vi "Test - DeviceManager - StartICL 1.vi"(8 "error in":errorcluster) -> (0 "error out":errorcluster, 3 "Pass":bool)   [LabVIEW 2023]
doc: "_____\nCreated using DQMH Event Scripter 7.0.0.1280."
uses:
  Source/Libraries/DeviceManager/DeviceManager.lvlib
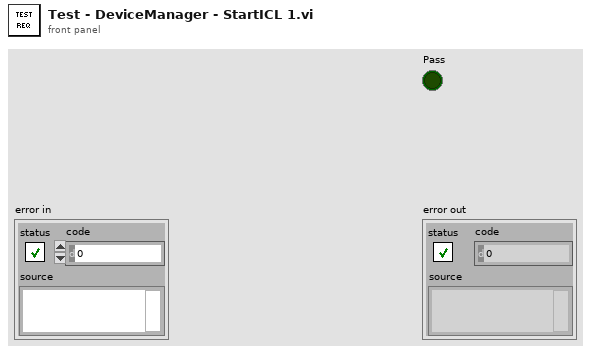
[diagram p1: front panel]
types:
  T1 = typedef "DeviceManager.lvlib/Broadcast Events--cluster.ctl" = cluster{"Module Did Init":refnum<user-event>, "Status Updated":refnum<user-event>, "Error Reported":refnum<user-event>, "Module Did Stop":refnum<user-event>, "Update Module Execution Status":refnum<user-event>}
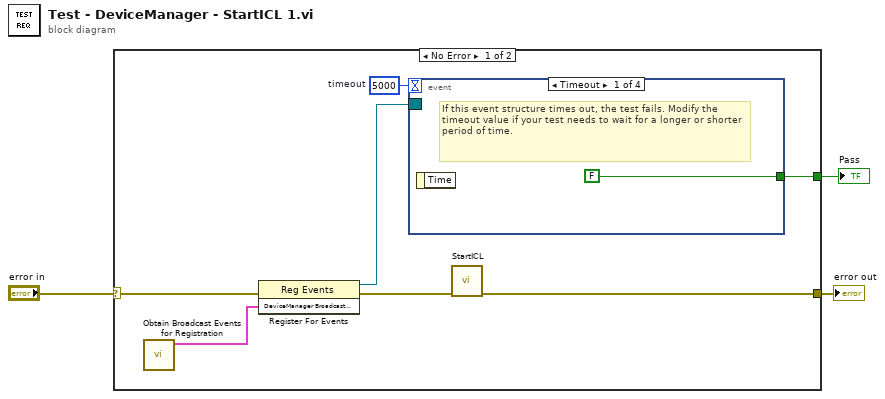
[diagram p0: block diagram]
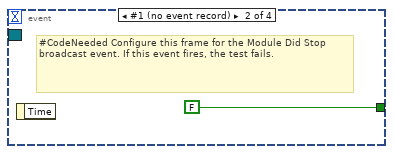
[diagram p2: hidden frame]
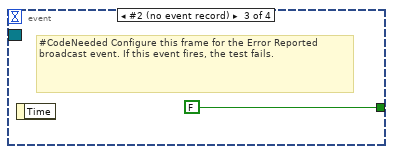
[diagram p3: hidden frame]
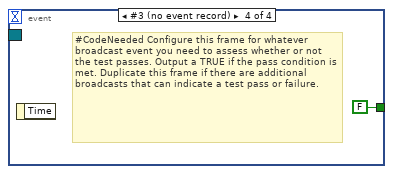
[diagram p4: hidden frame]
diagram:
  n1 = case shown="No Error" "error in" {
    selector: "error in" -> [w10 w15]
    tunnel: [w9 w15] -> w2
    tunnel: [w4 _] -> w1
    frame No Error {
      w5 = 5000  # timeout
      n2 = call "Obtain Broadcast Events for Registration.vi"() -> ("DeviceManager Broadcast Events"=w7:T1)  [unwired: 9 in, 2 out]
      n3 = register-events(error in=w10, w7) -> (reference out=w6:refnum<event-registration>, error out=w8:errorcluster)  [unwired: 1 in]
      n4 = event shown="[0] Timeout" {
        selector: w6 -> [_ _ _ _]
        dyn-events: _ -> [_ _ _ _]
        timeout: w5 -> [_ _ _ _]
        tunnel: [FALSE FALSE FALSE FALSE] -> w4
        event Timeout {
          # "If this event structure times out, the test fails. Modify the timeout value if your test needs to wait for a longer or shorter period of time."
          n5 = event-data() -> ()  [unwired: 1 in, 1 out]
        }
        event #1 (no event record) {
          # "#CodeNeeded Configure this frame for the Module Did Stop broadcast event. If this event fires, the test fails."
          n6 = event-data() -> ()  [unwired: 1 in, 1 out]
        }
        event #2 (no event record) {
          # "#CodeNeeded Configure this frame for the Error Reported broadcast event. If this event fires, the test fails."
          n7 = event-data() -> ()  [unwired: 1 in, 1 out]
        }
        event #3 (no event record) {
          # "#CodeNeeded Configure this frame for whatever broadcast event you need to assess whether or not the test passes. Output a TRUE if the pass condition is met. Duplicate this frame if there are additional broadcasts that can indicate a test pass or failure."
          n8 = event-data() -> ()  [unwired: 1 in, 1 out]
        }
      }
      n9 = call "StartICL.vi"("error in"=w8) -> ("error out"=w9:errorcluster)  [unwired: 10 in]
    }
    frame Error {
    }
  }
  "error out" <- w2
  "Pass" <- w1
